vi "Register gRPC Methods.vi"(8 "error in (no error)":errorcluster, 11 "Template Server in":refnum<class "PluginCore.lvclass">) -> (0 "error out":errorcluster, 3 "Template Server out":refnum<class "PluginCore.lvclass">)   [LabVIEW 2021, in "CIF_Plugin_Core_server.lvlib" / "PluginCore.lvclass"]
uses:
  PluginCore.lvclass
  typeDefs/Server Internal UEs.ctl
  typeDefs/Server Internal Message.ctl
  typeDefs/Server gRPC UEs.ctl
  <vilib>/gRPC/LabVIEW gRPC Library/Server API/typeDefs/gRPCId Cluster.ctl
  <vilib>/gRPC/LabVIEW gRPC Library/Shared/grpcId.ctl
  PluginCore.lvclass/PluginCore.ctl
  <vilib>/gRPC/LabVIEW gRPC Library/grpc-lvsupport-release.lvlib
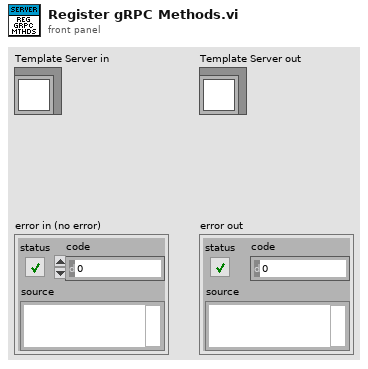
[diagram p1: front panel]
types:
  T1 = typedef "CIF_Plugin_Core_server.lvlib/PluginCore.lvclass/Server gRPC UEs.ctl" = cluster{"PluginCore Start gRPC UE":refnum<user-event>, "PluginCore Pause gRPC UE":refnum<user-event>, "PluginCore Stop gRPC UE":refnum<user-event>, "PluginCore RefreshStatistics gRPC UE":refnum<user-event>, "PluginCore UpdateConfig gRPC UE":refnum<user-event>, "PluginCore GetStatusData gRPC UE":refnum<user-event>, "PluginCore GetVersion gRPC UE":refnum<user-event>, "PluginCore GetConfig gRPC UE":refnum<user-event>, "PluginCore GetOverrides gRPC UE":refnum<user-event>}
  T2 = typedef "CIF_Plugin_Core_server.lvlib/PluginCore.lvclass/Server Internal UEs.ctl" = cluster{"PluginCore Start Internal UE":refnum<user-event>, "PluginCore Pause Internal UE":refnum<user-event>, "PluginCore Stop Internal UE":refnum<user-event>, "PluginCore RefreshStatistics Internal UE":refnum<user-event>, "PluginCore UpdateConfig Internal UE":refnum<user-event>, "PluginCore GetStatusData Internal UE":refnum<user-event>, "PluginCore GetVersion Internal UE":refnum<user-event>, "PluginCore GetConfig Internal UE":refnum<user-event>, "PluginCore GetOverrides Internal UE":refnum<user-event>}
  T3 = typedef "grpc-lvsupport-release.lvlib/grpcId.ctl" = u64
  T4 = typedef "CIF_Plugin_Core_server.lvlib/PluginCore.lvclass/Server Internal Message UE.ctl" = refnum<user-event>
  T5 = typedef "grpc-lvsupport-release.lvlib/gRPCId Cluster UE.ctl" = refnum<user-event>
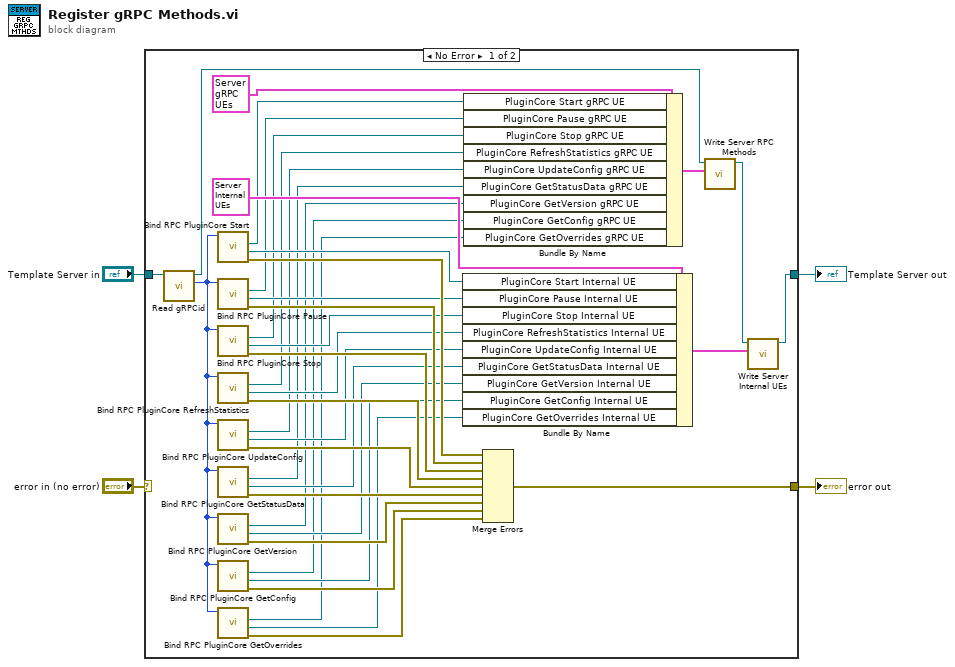
[diagram p0: block diagram]
diagram:
  n1 = case shown="No Error" "error in (no error)" {
    selector: "error in (no error)" -> [_ w42]
    tunnel: "Template Server in" -> [w33 w43]
    tunnel: [w41 w42] -> w3
    tunnel: [w40 w43] -> w2
    frame No Error {
      n2 = call-dynamic "Read gRPCid.vi"("iService in"=w33) -> ("gRPCid"=w32:T3, "iService out"=w34:refnum<class "PluginCore.lvclass">)  [unwired: 8 in, 1 out]
      n3 = call "Bind RPC PluginCore Start.vi"("gRPCid server in"=w32) -> ("error out"=w31:errorcluster, "PluginCore Start Internal UE"=w29:T4, "PluginCore Start gRPC UE"=w30:T5)  [unwired: 7 in, 1 out]
      n4 = call "Bind RPC PluginCore Pause.vi"("gRPCid server in"=w32) -> ("error out"=w28:errorcluster, "PluginCore Pause Internal UE"=w26:T4, "PluginCore Pause gRPC UE"=w27:T5)  [unwired: 7 in, 1 out]
      n5 = call "Bind RPC PluginCore Stop.vi"("gRPCid server in"=w32) -> ("error out"=w25:errorcluster, "PluginCore Stop Internal UE"=w23:T4, "PluginCore Stop gRPC UE"=w24:T5)  [unwired: 7 in, 1 out]
      n6 = call "Bind RPC PluginCore RefreshStatistics.vi"("gRPCid server in"=w32) -> ("error out"=w22:errorcluster, "PluginCore RefreshStatistics Internal UE"=w20:T4, "PluginCore RefreshStatistics gRPC UE"=w21:T5)  [unwired: 7 in, 1 out]
      n7 = call "Bind RPC PluginCore UpdateConfig.vi"("gRPCid server in"=w32) -> ("error out"=w19:errorcluster, "PluginCore UpdateConfig Internal UE"=w17:T4, "PluginCore UpdateConfig gRPC UE"=w18:T5)  [unwired: 7 in, 1 out]
      n8 = call "Bind RPC PluginCore GetStatusData.vi"("gRPCid server in"=w32) -> ("error out"=w16:errorcluster, "PluginCore GetStatusData Internal UE"=w14:T4, "PluginCore GetStatusData gRPC UE"=w15:T5)  [unwired: 7 in, 1 out]
      n9 = call "Bind RPC PluginCore GetVersion.vi"("gRPCid server in"=w32) -> ("error out"=w13:errorcluster, "PluginCore GetVersion Internal UE"=w11:T4, "PluginCore GetVersion gRPC UE"=w12:T5)  [unwired: 7 in, 1 out]
      n10 = call "Bind RPC PluginCore GetConfig.vi"("gRPCid server in"=w32) -> ("error out"=w10:errorcluster, "PluginCore GetConfig Internal UE"=w8:T4, "PluginCore GetConfig gRPC UE"=w9:T5)  [unwired: 7 in, 1 out]
      n11 = call "Bind RPC PluginCore GetOverrides.vi"("gRPCid server in"=w32) -> ("error out"=w7:errorcluster, "PluginCore GetOverrides Internal UE"=w5:T4, "PluginCore GetOverrides gRPC UE"=w6:T5)  [unwired: 7 in, 1 out]
      n12 = Bundle By Name ("Bundle Internal UEs")(cluster=T2 {"PluginCore Start Internal UE"=refnum, "PluginCore Pause Internal UE"=refnum, "PluginCore Stop Internal UE"=refnum, "PluginCore RefreshStatistics Internal UE"=refnum, "PluginCore UpdateConfig Internal UE"=refnum, "PluginCore GetStatusData Internal UE"=refnum, "PluginCore GetVersion Internal UE"=refnum, "PluginCore GetConfig Internal UE"=refnum, "PluginCore GetOverrides Internal UE"=refnum} ("Server Internal UEs"), "PluginCore Start Internal UE"=w29, "PluginCore Pause Internal UE"=w26, "PluginCore Stop Internal UE"=w23, "PluginCore RefreshStatistics Internal UE"=w20, "PluginCore UpdateConfig Internal UE"=w17, "PluginCore GetStatusData Internal UE"=w14, "PluginCore GetVersion Internal UE"=w11, "PluginCore GetConfig Internal UE"=w8, "PluginCore GetOverrides Internal UE"=w5) -> (w39:T2)
      n13 = Bundle By Name ("Bundle gRPC UEs")(cluster=T1 {"PluginCore Start gRPC UE"=refnum, "PluginCore Pause gRPC UE"=refnum, "PluginCore Stop gRPC UE"=refnum, "PluginCore RefreshStatistics gRPC UE"=refnum, "PluginCore UpdateConfig gRPC UE"=refnum, "PluginCore GetStatusData gRPC UE"=refnum, "PluginCore GetVersion gRPC UE"=refnum, "PluginCore GetConfig gRPC UE"=refnum, "PluginCore GetOverrides gRPC UE"=refnum} ("gRPC Server Method Events"), "PluginCore Start gRPC UE"=w30, "PluginCore Pause gRPC UE"=w27, "PluginCore Stop gRPC UE"=w24, "PluginCore RefreshStatistics gRPC UE"=w21, "PluginCore UpdateConfig gRPC UE"=w18, "PluginCore GetStatusData gRPC UE"=w15, "PluginCore GetVersion gRPC UE"=w12, "PluginCore GetConfig gRPC UE"=w9, "PluginCore GetOverrides gRPC UE"=w6) -> (w36:T1)
      n14 = Merge Errors(w31, w28, w25, w22, w19, w16, w13, w10, w7) -> (w41:errorcluster)
      n15 = call "Write Server RPC Methods.vi"("Server RPC Methods"=w36, "SignalGeneratorService in"=w34) -> ("SignalGeneratorService out"=w37:refnum<class "PluginCore.lvclass">)  [unwired: 8 in, 1 out]
      n16 = call "Write Server Internal UEs.vi"("Server Internal UEs"=w39, "SignalGeneratorService in"=w37) -> ("SignalGeneratorService out"=w40:refnum<class "PluginCore.lvclass">)  [unwired: 8 in, 1 out]
    }
    frame Error {
    }
  }
  "error out" <- w3
  "Template Server out" <- w2
